vi "data_file.vi"(4 "Nota 01":string, 8 "Sample name":string, 11 "File name":string) -> (0 "path":path)   [LabVIEW 2011]
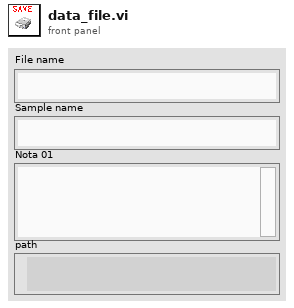
[diagram p1: front panel]
types:
  T1 = enum16{"open", "replace", "create", "open or create", "replace or create", "replace or create with confirmation"}
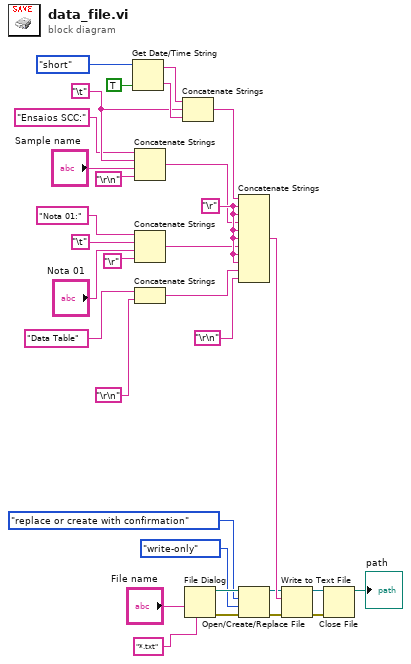
[diagram p0: block diagram]
diagram:
  w22 = "\r"
  w5 = "\t"
  n1 = Get Date/Time String(date format (0)=enum16{"short", "long", "abbreviated"}."short", want seconds? (F)=TRUE) -> (date string=w28:string, time string=w27:string)  [unwired: 1 in]
  n2 = Concatenate Strings("Ensaios SCC:" ("string"), w5, "Sample name", "\r\n") -> (w3:string)
  n3 = Concatenate Strings("Nota 01:" ("Nota 4"), "\t", "Nota 01", "\r") -> (w18:string)
  n4 = Concatenate Strings("Data Table" ("string"), "\r\n") -> (w23:string)
  n5 = Concatenate Strings(w28, w5, w27) -> (w24:string)
  n6 = File Dialog(6:"*.txt" ("pattern label"), 9:"File name") -> (0:w16:errorcluster, 3:w17:path)  [unwired: 2 in, 5 out]
  n7 = Concatenate Strings(w24, w22, w22, w3, w22, w22, w18, w22, w22, w23, "\r\n") -> (w26:string)
  n8 = Open/Create/Replace File(file path (use dialog)=w17, error in=w16, operation (0:open)=T1."replace or create with confirmation", access (0:read/write)=enum16{"read/write", "read-only", "write-only"}."write-only") -> (refnum out=w13:refnum<file>, error out=w12:errorcluster)  [unwired: 3 out]
  n9 = Write to Text File(file (use dialog)=w13, text=w26, error in=w12) -> (refnum out=w11:refnum<file>, error out=w8:errorcluster)  [unwired: 1 in, 1 out]
  n10 = Close File(refnum=w11, error in=w8) -> (path=→"path":path)  [unwired: 1 out]
